vi "stop.vi"(8 "error in (no error)":errorcluster, 11 "DAQ_DL090211Scaffold in":refnum<class "DAQ_DL090211Scaffold.lvclass">) -> (0 "error out":errorcluster, 3 "DAQ_DL090211Scaffold out":refnum<class "DAQ_DL090211Scaffold.lvclass">)   [LabVIEW 2010, in "DAQ_DL090211Scaffold.lvclass"]
uses:
  DAQ_DL090211Scaffold.lvclass
  GenericDAQ/GenericDAQ/GenericDAQ.lvclass
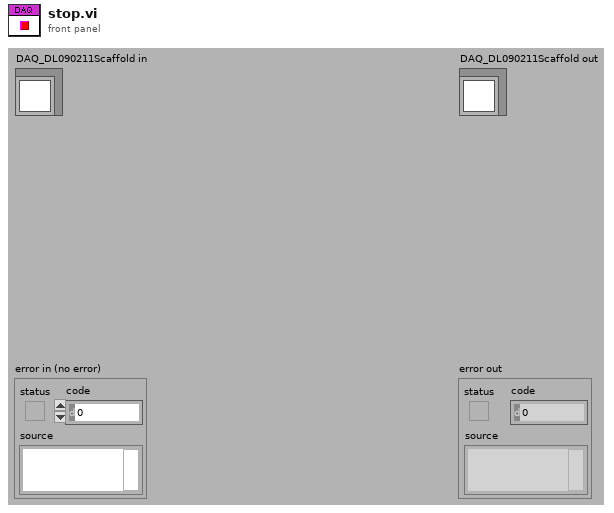
[diagram p1: front panel]
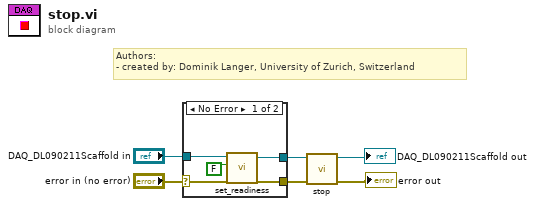
[diagram p0: block diagram]
diagram:
  # "Authors: \n- created by: Dominik Langer, University of Zurich, Switzerland"
  n1 = case shown="No Error" "error in (no error)" {
    selector: "error in (no error)" -> [w10 w13]
    tunnel: [w9 w13] -> w2
    tunnel: [w7 w12] -> w1
    tunnel: "DAQ_DL090211Scaffold in" -> [w8 w12]
    frame No Error {
      n2 = call-dynamic "set_readiness.vi"("error in (no error)"=w10, "ready?"=FALSE, "DAQ_DL090211Scaffold in"=w8) -> ("error out"=w9:errorcluster, "DAQ_DL090211Scaffold out"=w7:refnum<class "DAQ_DL090211Scaffold.lvclass">)  [unwired: 7 in]
    }
    frame Error {
    }
  }
  n3 = call-parent "stop.vi"("error in (no error)"=w2, "GenericToplevelComponent in"=w1) -> ("error out"=→"error out":errorcluster, "GenericToplevelComponent out"=→"DAQ_DL090211Scaffold out":refnum<class "DAQ_DL090211Scaffold.lvclass">)  [unwired: 8 in]
